vi "Label Targets Ball.vi"(5 "Details":bool, 6 "Color":u32(colorbox)=786176, 7 "Annotate":bool=TRUE, 8 "Score Threshold":dbl, 9 "results":T1, 10 "Angle":dbl=53.2 format="%#_13g", 11 "Image in":T2) -> (3 "Image out":T2)   [LabVIEW 2023]
doc: "Draw scores near or on the particle and an ellipse around the target. Scores that are below the score threshold are drawn in red, above in green."
uses:
  <vilib>/vision/Image Controls.llb/IMAQ Image.ctl
  Target Fields.ctl
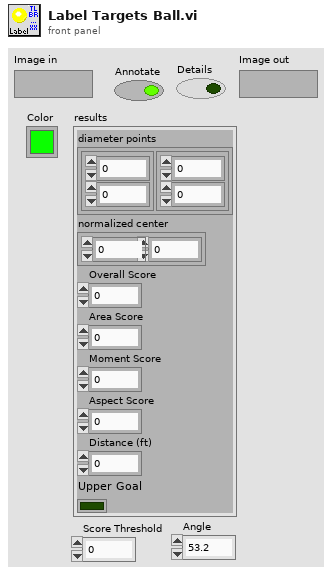
[diagram p1: front panel]
types:
  T1 = typedef "Target Fields.ctl" = cluster{"diameter points":cluster{"first point":cluster{"x":dbl, "y":dbl}, "projected point":cluster{"x":dbl, "y":dbl}}, "normalized center":cluster{"x":dbl, "y":dbl}, "Overall Score":dbl, "Area Score":dbl, "Moment Score":dbl, "Aspect Score":dbl, "Distance (ft)":dbl, "Upper Goal":bool}
  T2 = typedef "IMAQ Image.ctl" = refnum<image>
  T3 = cluster{"Desired Font (Application)":enum16{"User-specified Font", "Application Font", "System Font", "Dialog Font"}, "[User-specified Font]":cluster{"Font Name":string, "Size":i16, "Strikeout?":bool, "Italic?":bool, "Underline?":bool, "Outline?":bool, "Shadow?":bool, "Bold?":bool, "Rotation Angle":dbl}, "Horizontal Alignment":i16, "Vertical Alignment":i16}
  T4 = cluster{"first point":cluster{"x":dbl, "y":dbl}, "projected point":cluster{"x":dbl, "y":dbl}}
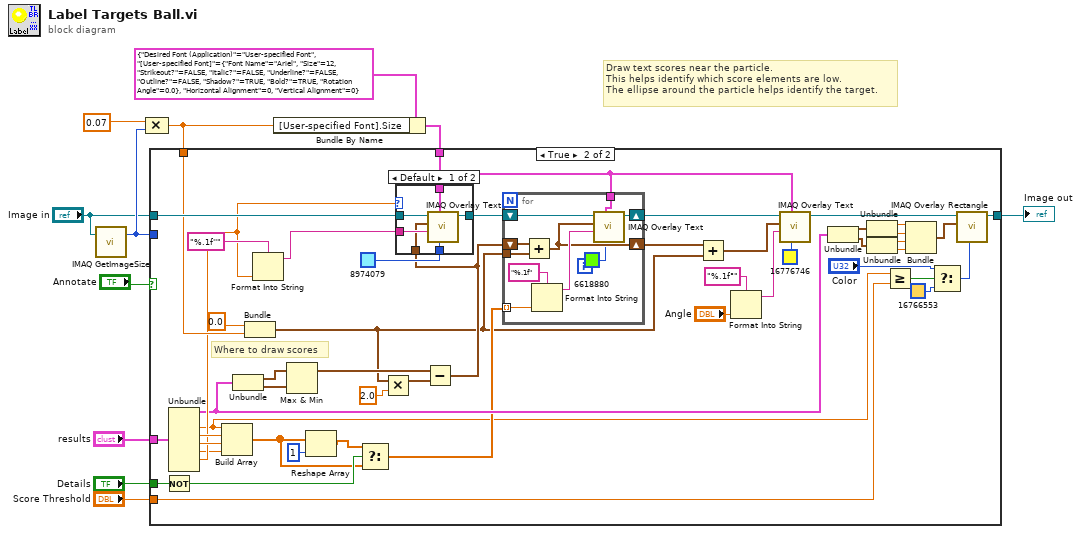
[diagram p0: block diagram]
diagram:
  # "Draw text scores near the particle.\nThis helps identify which score elements are low.\nThe ellipse around the particle helps identify the target."
  n1 = call "IMAQ GetImageSize"("Image"="Image in") -> ("Y Resolution"=w8:i32)  [unwired: 3 in, 2 out]
  n2 = Compound Arithmetic op=MULTIPLY(0.07, w8) -> (w5:dbl)
  n3 = Bundle By Name(cluster=T3 {"Desired Font (Application)"=enum."User-specified Font", "[User-specified Font]"={"Font Name"="Ariel", "Size"=12, "Strikeout?"=FALSE, "Italic?"=FALSE, "Underline?"=FALSE, "Outline?"=FALSE, "Shadow?"=TRUE, "Bold?"=TRUE, "Rotation Angle"=0.0}, "Horizontal Alignment"=0, "Vertical Alignment"=0} ("Font, Size & Style"), "[User-specified Font].Size"=w5) -> (w6:T3)
  n4 = case shown="True" "Annotate" {
    tunnel: [w12 w55] -> w11
    tunnel: "Image in" -> [w12 w61]
    tunnel: w6 -> [_ w20]
    tunnel: w8 -> [_ _]
    tunnel: w5 -> [_ w57]
    tunnel: "results" -> [_ w56]
    tunnel: "Score Threshold" -> [_ w28]
    tunnel: "Details" -> [_ w38]
    frame False {
    }
    frame True {
      # "Where to draw scores"
      n5 = Not(x=w38) -> (.not. x?=w37:bool)
      n6 = Unbundle(w56) -> ("diameter points"=w46:T4, "Overall Score"=w27:dbl, "Area Score"=w54:dbl, "Moment Score"=w50:dbl, "Aspect Score"=w47:dbl, "Distance (ft)"=w48:dbl)  [unwired: 2 out]
      n7 = Build Array(w27, w54, w50, w47) -> (w35:dbl[])
      n8 = Unbundle(w46) -> ("first point"=w51:cluster{"x":dbl, "y":dbl}, "projected point"=w52:cluster{"x":dbl, "y":dbl})
      n9 = Bundle(0.0, w57) -> (w15:cluster{dbl, dbl})  [unwired: 1 in]
      n10 = Format Into String(format string="%.1f''", w48) -> (resulting string=w60:string)  [unwired: 2 in, 1 out]
      n11 = Max & Min(x=w51, y=w52) -> (max(x,y)=w16:cluster{"x":dbl, "y":dbl})  [unwired: 1 out]
      n12 = Reshape Array(w35, 1) -> (w36:dbl[])
      n13 = Select(t=w36, s=w37, f=w35) -> (s? t:f=w34:dbl[])
      n14 = Multiply(x=w15, y=2.0) -> (x*y=w14:cluster{dbl, dbl})
      n15 = Subtract(x=w16, y=w14) -> (x-y=w17:cluster{dbl, dbl})
      n16 = case shown="Default" w48 {
        tunnel: w61 -> [w77 w78]
        tunnel: w60 -> [w76 _]
        tunnel: w20 -> [w75 _]
        tunnel: [w74 w78] -> w53
        tunnel: w17 -> [w73 _]
        tunnel: u32 8974079 ("Color") -> [w72 _]
        frame Default {
          n17 = call "IMAQ Overlay Text"("Text Color (black)"=w72, "Font, Size & Style"=w75, "String"=w76, "Origin"=w73, "Image"=w77) -> ("Image Out"=w74:T2)  [unwired: 5 in, 1 out]
        }
        frame 0 {
        }
      }
      n18 = for {
        tunnel: w34 -> [w62] mode=indexing
        shift-right: [w68] -> w24
        shift-left: w53 -> [w69]
        tunnel: w20 -> [w67]
        shift-right: [w64] -> w19
        shift-left: w17 -> [w65]
        tunnel: w15 -> [w66]
        n19 = Add(x=w65, y=w66) -> (x+y=w64:cluster{dbl, dbl})
        n20 = Format Into String(format string="%.1f", w62) -> (resulting string=w70:string)  [unwired: 2 in, 1 out]
        n21 = call "IMAQ Overlay Text"("Text Color (black)"=u32 6618880 ("Color"), "Font, Size & Style"=w67, "String"=w70, "Origin"=w64, "Image"=w69) -> ("Image Out"=w68:T2)  [unwired: 5 in, 1 out]
      }
      n22 = Add(x=w19, y=w15) -> (x+y=w18:cluster{dbl, dbl})
      n23 = Format Into String(format string="%.1f°", "Angle") -> (resulting string=w25:string)  [unwired: 2 in, 1 out]
      n24 = call "IMAQ Overlay Text"("Text Color (black)"=u32 16776746 ("Color"), "Font, Size & Style"=w20, "String"=w25, "Origin"=w18, "Image"=w24) -> ("Image Out"=w23:T2)  [unwired: 5 in, 1 out]
      n25 = Unbundle(w46) -> ("first point"=w45:cluster{"x":dbl, "y":dbl}, "projected point"=w44:cluster{"x":dbl, "y":dbl})
      n26 = Unbundle(w45) -> ("x"=w43:dbl, "y"=w42:dbl)
      n27 = Unbundle(w44) -> ("x"=w41:dbl, "y"=w40:dbl)
      n28 = Greater Or Equal?(x=w27, y=w28) -> (x >= y?=w29:bool)
      n29 = Bundle("x"=w43, "y"=w42, "x"=w41, "y"=w40) -> (w39:cluster{"x":dbl, "y":dbl, "x":dbl, "y":dbl})  [unwired: 1 in]
      n30 = Select(t="Color", s=w29, f=u32 16766553 ("Color")) -> (s? t:f=w30:u32)
      n31 = call "IMAQ Overlay Rectangle"("Color"=w30, "Rectangle"=w39, "Image"=w23) -> ("Image Out"=w55:T2)  [unwired: 7 in, 1 out]
    }
  }
  "Image out" <- w11
